vi "OAT Demodulation with Decimation (1 Freq, 1 Ch).vi"(0 "x[n]":dbl[](array[numeric]) format="%.2f", 1 "reset? (True)":bool=TRUE, 2 "zero delay? (F)":bool, 5 "fs":dbl=1.0 format="%.2f", 9 "fc [Hz]":dbl format="%.2f", 11 "decimation factor":i32=16, 12 "stop band attenuation":u16(ring) items=["72 dB", "96 dB", "120 dB"], 14 "phase setting":T1) -> (4 "magnitudes":dbl[](array[numeric]) format="%.2f", 6 "phases":dbl[](array[numeric]) format="%.2f", 10 "new fs [Hz]":dbl format="%.2f", 15 "error out":errorcluster)   [LabVIEW 2017, in "SoundVib_Resampling.lvlib"]
uses:
  <vilib>/addons/Sound and Vibration/Order Analysis/Resample Order Tracking/SoundVib_Resampling.lvlib
panel:
  # "Demodulation"
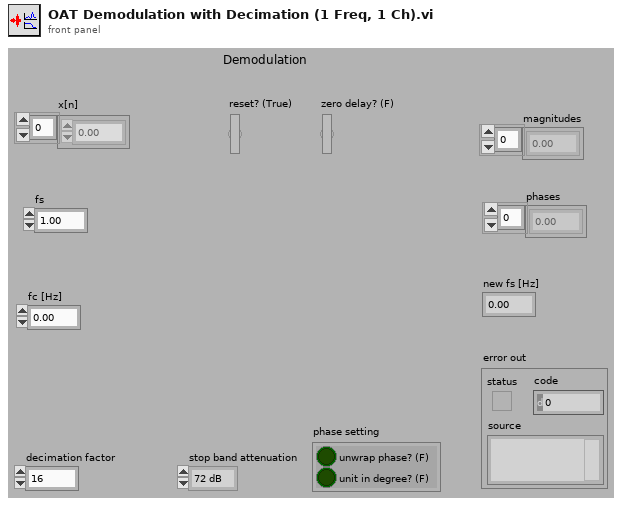
[diagram p1: front panel]
types:
  T1 = cluster{"unwrap phase? (F)":bool, "unit in degree? (F)":bool}
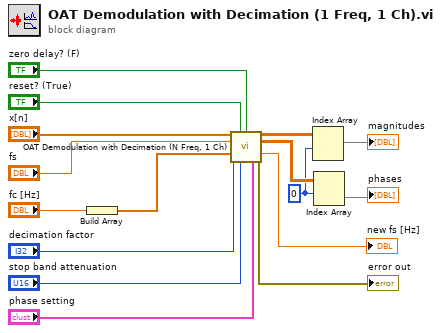
[diagram p0: block diagram]
diagram:
  w6 = 0 ("index (row)")
  n1 = Build Array("fc [Hz]") -> (w13:dbl[])
  n2 = call <vilib>:"OAT Demodulation with Decimation (N Freq, 1 Ch).vi"("x[n]"="x[n]", "reset? (True)"="reset? (True)", "zero delay? (F)"="zero delay? (F)", "fs"="fs", "fc [Hz]"=w13, "decimation factor"="decimation factor", "stop band attenuation"="stop band attenuation", "phase setting"="phase setting") -> ("magnitudes (RMS)"=w10:dbl[][], "phase lag"=w8:dbl[][], "new fs [Hz]"=→"new fs [Hz]":dbl, "error out"=→"error out":errorcluster)  [unwired: 3 in, 1 out]
  n3 = Index Array(array=w10, index (row)=w6) -> (element=→"magnitudes":dbl[])  [unwired: 1 in]
  n4 = Index Array(array=w8, index (row)=w6) -> (element=→"phases":dbl[])  [unwired: 1 in]
